vi "ReadWrite config.vi"(6 "Config":T2, 8 "error in (no error)":errorcluster, 9 "Mail Server in":T1={"Outgoing Mail Server (SMTP)"="smtp.gmail.com", "MAIL Account User ID"="who", "MAIL Account Password"="", "Enable SSL"=TRUE, "Port"=587, "Sender's Email Address"="who@gmail.com", "Sender's Name"="first last"}, 10 "SVN in":T3, 11 "Paths in":T4) -> (0 "error out":errorcluster, 1 "Mail Server":T1={"Outgoing Mail Server (SMTP)"="smtp.gmail.com", "MAIL Account User ID"="monroews", "MAIL Account Password"="", "Enable SSL"=TRUE, "Port"=587, "Sender's Email Address"="monroews@gmail.com", "Sender's Name"="Monroe Weber-Shirk"}, 2 "SVN":T3, 3 "Paths":T4)   [LabVIEW 2012]
uses:
  Paths.ctl
  SVN.ctl
  Folders.ctl
  ReadWrite.ctl
  Mail Server.ctl
  <vilib>/Utility/config.llb/Read Key (Path).vi
  <vilib>/Utility/config.llb/Write Key (Path).vi
  <vilib>/Utility/config.llb/Write Key (String).vi
  <vilib>/Utility/config.llb/Read Key (String).vi
  Design Server.lvlib
  <vilib>/Utility/config.llb/NI_LVConfig.lvlib
panel:
  in  "Folders":T5
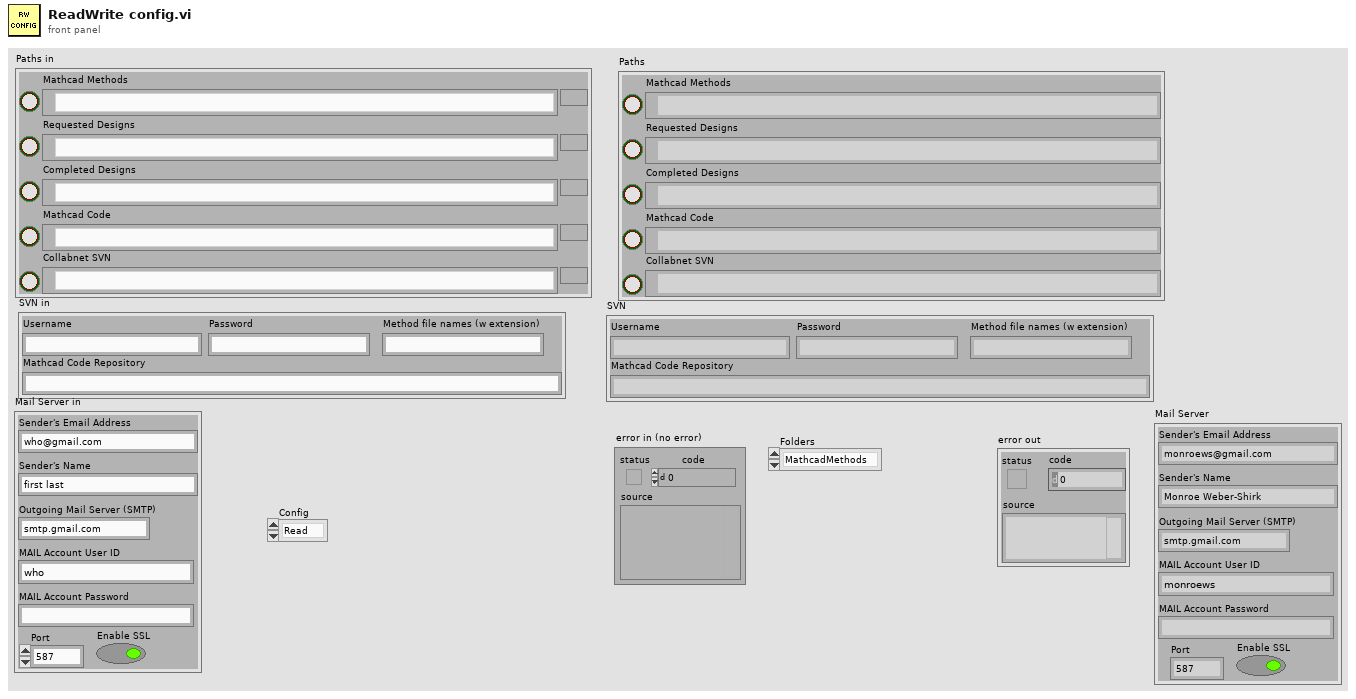
[diagram p1: front panel]
types:
  T1 = typedef "Mail Server.ctl" = cluster{"Outgoing Mail Server (SMTP)":string, "MAIL Account User ID":string, "MAIL Account Password":string, "Enable SSL":bool, "Port":i32, "Sender's Email Address":string, "Sender's Name":string}
  T2 = typedef "ReadWrite.ctl" = enum16{"Read", "Write"}
  T3 = typedef "SVN.ctl" = cluster{"Mathcad Code Repository":string, "Username":string, "Password":string, "Method file names (w extension)":string}
  T4 = typedef "Paths.ctl" = cluster{"Mathcad Methods":path, "Requested Designs":path, "Completed Designs":path, "Mathcad Code":path, "Collabnet SVN":path, "Mathcad Methods ok":bool, "Requested Designs ok":bool, "Completed Designs ok":bool, "Mathcad Code ok":bool, "Collabnet SVN":bool}
  T5 = typedef "Design Server.lvlib/Folders.ctl" = enum16{"MathcadMethods", "RequestedDesigns", "CompletedDesigns", "MathcadCode", "CollabnetSVN.exe"}
  T6 = cluster{"[0]":string, "[1]":string, "[2]":string, "[3]":string}
  T7 = typedef "NI_LVConfig.lvlib/Config Data RefNum.ctl" = refnum<k1>
  T8 = cluster{"[0]":path, "[1]":path, "[2]":path, "[3]":path, "[4]":path}
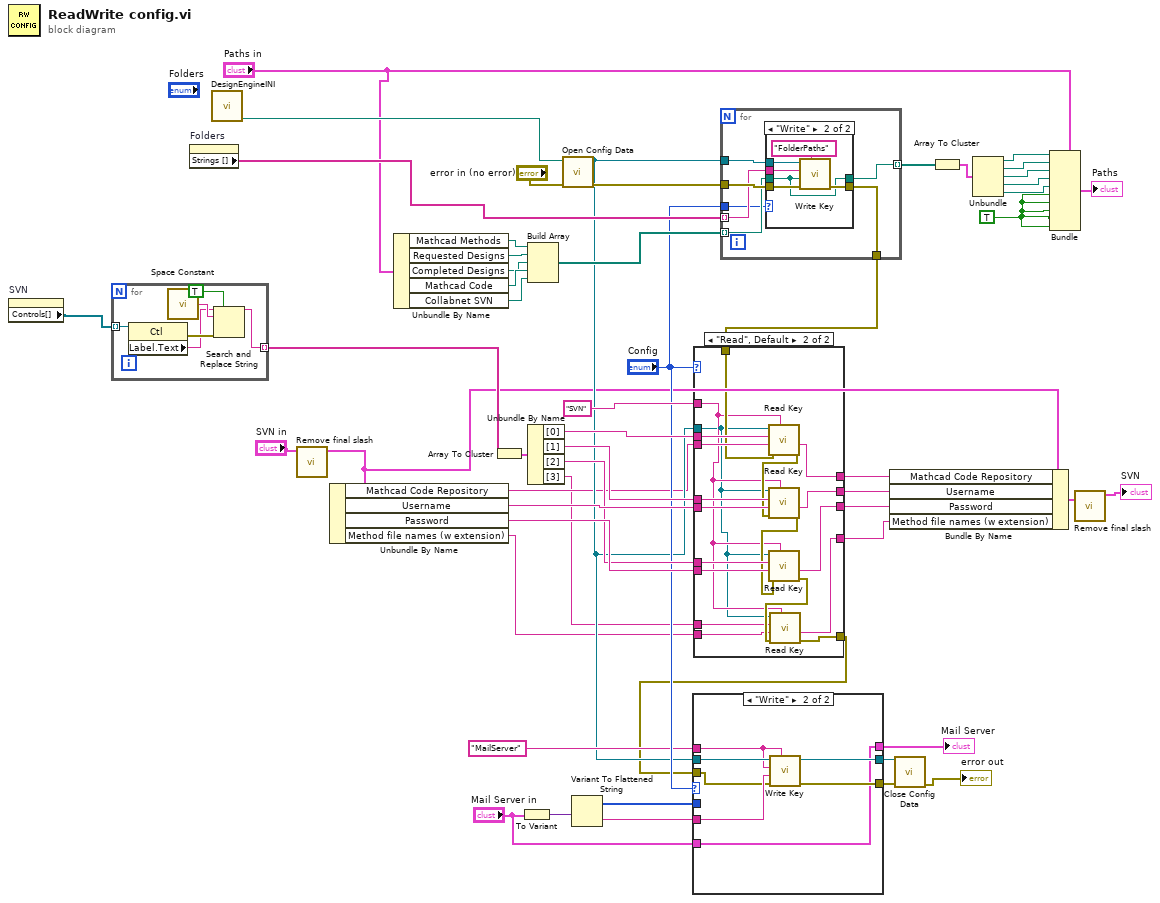
[diagram p0: block diagram]
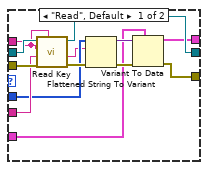
[diagram p2: hidden frame]
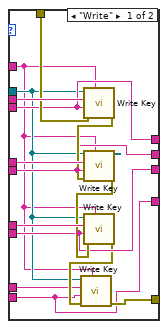
[diagram p3: hidden frame]
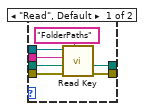
[diagram p4: hidden frame]
diagram:
  w20 = TRUE ("Mathcad Methods ok")
  n1 = property on="SVN" class="Clust (strict)"() -> ("Controls[]"=w31:refnum<vi>[])  [unwired: 2 in, 2 out]
  n2 = for {
    tunnel: w31 -> [w59] mode=indexing
    tunnel: [w55] -> w41 mode=indexing
    n3 = property class="Ctl"(reference=w59) -> (error out=w58:errorcluster, "Label.Text"=w56:string)  [unwired: 1 in, 1 out]
    n4 = call <vilib>:"Space Constant.vi"() -> ("String"=w57:string)
    n5 = Search and Replace String(replace all?=TRUE ("replace all? (F)"), input string=w56, search string=w57, error in=w58) -> (result string=w55:string)  [unwired: 4 in, 3 out]
  }
  n6 = property on="Folders" class="Enum (strict)"() -> ("Strings []"=w34:string[])  [unwired: 2 in, 2 out]
  n7 = call "DesignEngineINI.vi"() -> ("Ini file path"=w47:path)  [unwired: 6 in, 1 out]
  n8 = call "Remove final slash.vi"("SVN"="SVN in") -> ("SVN out"=w7:T3)  [unwired: 10 in]
  n9 = Unbundle By Name(w7) -> ("Mathcad Code Repository"=w6:string, "Username"=w44:string, "Password"=w43:string, "Method file names (w extension)"=w2:string)
  n10 = Unbundle By Name("Paths in") -> ("Mathcad Methods"=w24:path, "Requested Designs"=w25:path, "Completed Designs"=w26:path, "Mathcad Code"=w27:path, "Collabnet SVN"=w22:path)
  n11 = Array To Cluster(array=w41) -> (cluster=w40:T6)
  n12 = To Variant(anything="Mail Server in") -> (Variant=w16:variant)
  n13 = Build Array(w24, w25, w26, w27, w22) -> (w23:path[])
  n14 = Unbundle By Name(w40) -> ("[0]"=w39:string, "[1]"=w38:string, "[2]"=w37:string, "[3]"=w3:string)
  n15 = call <vilib>:"Open Config Data.vi"("error in (no error)"="error in (no error)", "configuration file path"=w47) -> ("error out"=w46:errorcluster, "refnum"=w17:T7)  [unwired: 7 in, 1 out]
  n16 = Variant To Flattened String(Variant=w16) -> (data string=w15:string, 1:w11:i16[])
  n17 = for {
    tunnel: w46 -> [w66]
    tunnel: w17 -> [w65]
    tunnel: w34 -> [w64] mode=indexing
    tunnel: w23 -> [w63] mode=indexing
    tunnel: [w62] -> w48 mode=indexing
    tunnel: [w61] -> w33
    tunnel: "Config" -> [w60]
    n18 = case shown="\"Write\"" w60 {
      tunnel: w66 -> [w72 w78]
      tunnel: w65 -> [w71 w77]
      tunnel: w64 -> [w70 w76]
      tunnel: w63 -> [w69 w74]
      tunnel: [w68 w74] -> w62
      tunnel: [w67 w75] -> w61
      frame "Read", Default {
        n19 = call-poly <vilib>:"Read Key.vi"("section"="FolderPaths", "error in (no error)"=w72, "default value"=w69, "key"=w70, "refnum"=w71) -> ("error out"=w67:errorcluster, "value"=w68:path)  [unwired: 3 in, 2 out]
      }
      frame "Write" {
        n20 = call-poly <vilib>:"Write Key.vi"("section"="FolderPaths", "error in (no error)"=w78, "value"=w74, "key"=w76, "refnum"=w77) -> ("error out"=w75:errorcluster)  [unwired: 4 in, 2 out]
      }
    }
  }
  n21 = case shown="\"Read\", Default" "Config" {
    tunnel: w6 -> [w88 w113]
    tunnel: w44 -> [w87 w112]
    tunnel: w43 -> [w86 w111]
    tunnel: w17 -> [w83 w95]
    tunnel: "SVN" ("section") -> [w82 w96]
    tunnel: w39 -> [w94 w110]
    tunnel: w38 -> [w93 w109]
    tunnel: w37 -> [w92 w108]
    tunnel: [w88 w107] -> w36
    tunnel: [w87 w106] -> w35
    tunnel: w33 -> [w91 w105]
    tunnel: [w85 w100] -> w14
    tunnel: [w86 w102] -> w30
    tunnel: w3 -> [w81 w98]
    tunnel: w2 -> [w80 w97]
    tunnel: [w80 w99] -> w1
    frame "Write" {
      n22 = call-poly <vilib>:"Write Key.vi"("section"=w82, "error in (no error)"=w91, "value"=w88, "key"=w94, "refnum"=w83) -> ("error out"=w90:errorcluster)  [unwired: 4 in, 2 out]
      n23 = call-poly <vilib>:"Write Key.vi"("section"=w82, "error in (no error)"=w90, "value"=w87, "key"=w93, "refnum"=w83) -> ("error out"=w89:errorcluster)  [unwired: 4 in, 2 out]
      n24 = call-poly <vilib>:"Write Key.vi"("section"=w82, "error in (no error)"=w89, "value"=w86, "key"=w92, "refnum"=w83) -> ("error out"=w84:errorcluster)  [unwired: 4 in, 2 out]
      n25 = call-poly <vilib>:"Write Key.vi"("section"=w82, "error in (no error)"=w84, "value"=w80, "key"=w81, "refnum"=w83) -> ("error out"=w85:errorcluster)  [unwired: 4 in, 2 out]
    }
    frame "Read", Default {
      n26 = call-poly <vilib>:"Read Key.vi"("section"=w96, "error in (no error)"=w105, "default value"=w113, "key"=w110, "refnum"=w95) -> ("error out"=w104:errorcluster, "value"=w107:string)  [unwired: 3 in, 2 out]
      n27 = call-poly <vilib>:"Read Key.vi"("section"=w96, "error in (no error)"=w104, "default value"=w112, "key"=w109, "refnum"=w95) -> ("error out"=w103:errorcluster, "value"=w106:string)  [unwired: 3 in, 2 out]
      n28 = call-poly <vilib>:"Read Key.vi"("section"=w96, "error in (no error)"=w103, "default value"=w111, "key"=w108, "refnum"=w95) -> ("error out"=w101:errorcluster, "value"=w102:string)  [unwired: 3 in, 2 out]
      n29 = call-poly <vilib>:"Read Key.vi"("section"=w96, "error in (no error)"=w101, "default value"=w97, "key"=w98, "refnum"=w95) -> ("error out"=w100:errorcluster, "value"=w99:string)  [unwired: 3 in, 2 out]
    }
  }
  n30 = case shown="\"Write\"" "Config" {
    tunnel: "MailServer" ("section") -> [w124 w132]
    tunnel: w17 -> [w125 w133]
    tunnel: w15 -> [w123 w131]
    tunnel: w14 -> [w126 w130]
    tunnel: [w118 w129] -> w13
    tunnel: [w120 w128] -> w12
    tunnel: w11 -> [w117 _]
    tunnel: "Mail Server in" -> [w115 w127]
    tunnel: [w114 w127] -> w9
    frame "Read", Default {
      n31 = call-poly <vilib>:"Read Key.vi"("section"=w124, "error in (no error)"=w126, "default value"=w123, "key"=w124, "refnum"=w125) -> ("error out"=w119:errorcluster, "value"=w116:string, "refnum out"=w120:T7)  [unwired: 3 in, 1 out]
      n32 = Flattened String To Variant(4:w119, 6:w116, 7:w117) -> (0:w121:errorcluster, 3:w122:variant)
      n33 = Variant To Data(error in=w121, type=w115, Variant=w122) -> (data=w114:T1, error out=w118:errorcluster)
    }
    frame "Write" {
      n34 = call-poly <vilib>:"Write Key.vi"("section"=w132, "error in (no error)"=w130, "value"=w131, "key"=w132, "refnum"=w133) -> ("error out"=w129:errorcluster, "refnum out"=w128:T7)  [unwired: 4 in, 1 out]
    }
  }
  "Mail Server" <- w9
  n35 = Bundle By Name(cluster=w7, "Mathcad Code Repository"=w36, "Username"=w35, "Password"=w30, "Method file names (w extension)"=w1) -> (w5:T3)
  n36 = call <vilib>:"Close Config Data.vi"("error in (no error)"=w13, "refnum"=w12) -> ("error out"=→"error out":errorcluster)  [unwired: 8 in, 1 out]
  n37 = Array To Cluster(array=w48) -> (cluster=w49:T8)
  n38 = Unbundle(w49) -> ("[0]"=w50:path, "[1]"=w51:path, "[2]"=w52:path, "[3]"=w53:path, "[4]"=w21:path)
  n39 = Bundle(cluster="Paths in", "Mathcad Methods"=w50, "Requested Designs"=w51, "Completed Designs"=w52, "Mathcad Code"=w53, "Collabnet SVN"=w21, "Mathcad Methods ok"=w20, "Requested Designs ok"=w20, "Completed Designs ok"=w20, "Mathcad Code ok"=w20, "Collabnet SVN"=w20) -> (→"Paths":T4)
  n40 = call "Remove final slash.vi"("SVN"=w5) -> ("SVN out"=→"SVN":T3)  [unwired: 10 in]
